vi "Dialog Window.vi"(10 "Message":string, 11 "Title":string="HPS17K Panel Notification") -> ()   [LabVIEW 2023]
uses:
  <userlib>/_OpenG.lib/appcontrol/appcontrol.llb/openg_application_control.lvlib
panel:
  in  "OK":bool
  out "Time Stamp":timestamp format="%<%x %.3X>T"
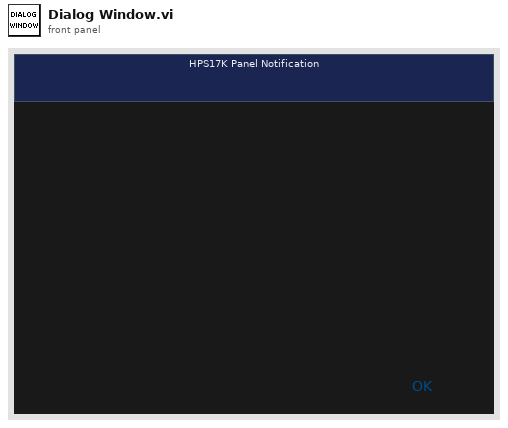
[diagram p1: front panel]
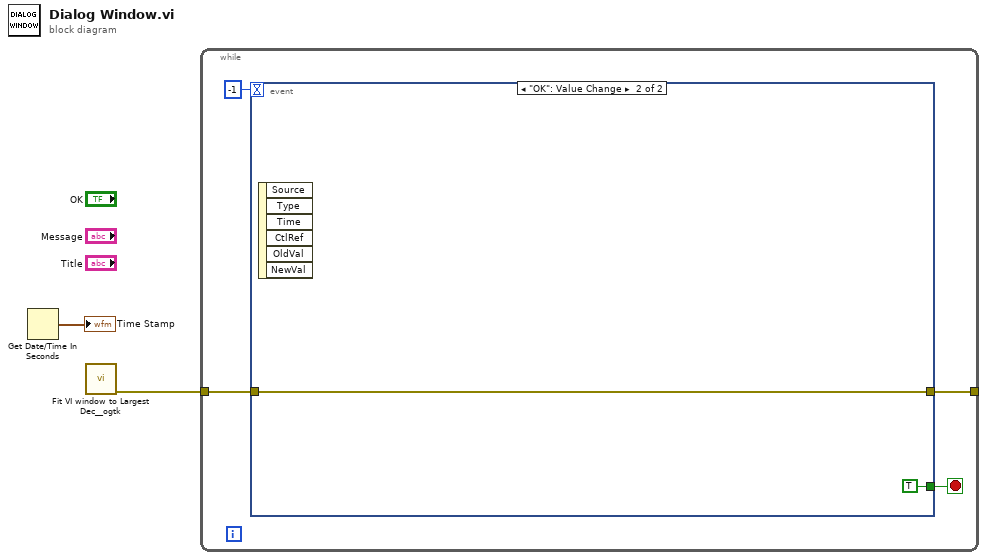
[diagram p0: block diagram]
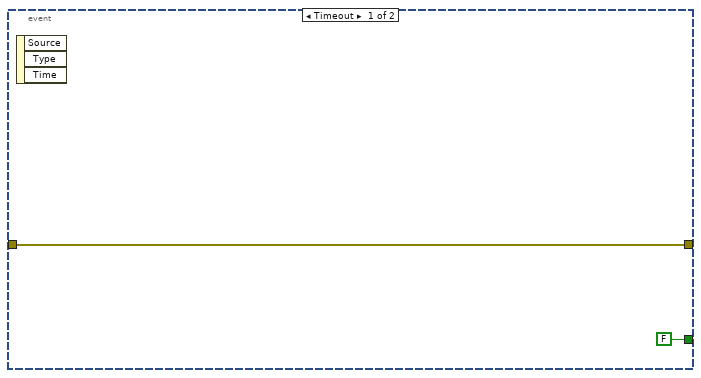
[diagram p2: hidden frame]
diagram:
  n1 = Get Date/Time In Seconds() -> (seconds since 1Jan1904=→"Time Stamp":timestamp)
  n2 = call <userlib>:"Fit VI window to Largest Dec__ogtk.vi"() -> ("error out"=w1:errorcluster)  [unwired: 6 in, 1 out]
  n3 = while {
    tunnel: w1 -> [w5]
    tunnel: [w4] -> _
    stop <- w3 stop-if-true
    n4 = event shown="[1] \"OK\": Value Change" {
      selector: _ -> [_ _]
      dyn-events: _ -> [_ _]
      timeout: -1 -> [_ _]
      tunnel: w5 -> [w8 w10]
      tunnel: [w8 w10] -> w4
      tunnel: [FALSE TRUE] -> w3
      event Timeout {
        n5 = event-data() -> ()  [unwired: 1 in, 3 out]
      }
      event "OK": Value Change {
        n6 = event-data() -> ()  [unwired: 1 in, 6 out]
      }
    }
  }
